vi "GLdrv_Read_USB.vi"(0 "hDevice":i32, 5 "Count":u32, 7 "Term(CrLf)":string="\r\n", 11 "error in (no error)":errorcluster, 12 "dwTimeOut":i32=1000) -> (4 "dup hDevice":i32, 6 "lpBuffer":string, 8 "lpNumberOfBytesRead":u32, 15 "error out":errorcluster)   [LabVIEW 2017]
uses:
  gtcusbr.dll
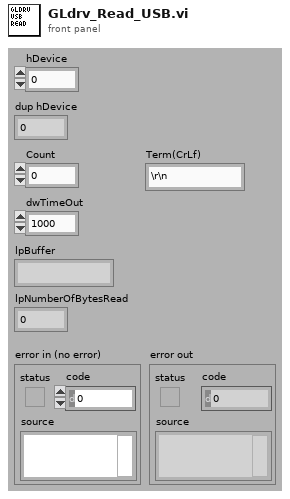
[diagram p1: front panel]
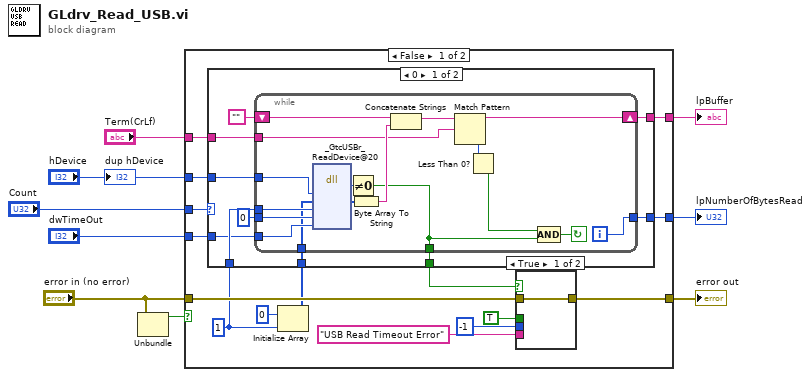
[diagram p0: block diagram]
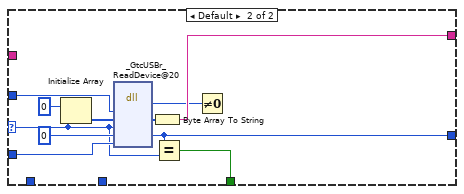
[diagram p2: hidden frame]
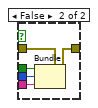
[diagram p3: hidden frame]
diagram:
  n1 = Unbundle("error in (no error)") -> ("status"=w4:bool)  [unwired: 2 out]
  n2 = case shown="FALSE" w4 {
    tunnel: "hDevice" -> [w24 _]
    tunnel: "dwTimeOut" -> [w23 _]
    tunnel: [w17 _] -> w7
    tunnel: [w16 _] -> w6
    tunnel: "error in (no error)" -> [w19 w69]
    tunnel: [w20 w69] -> w3
    tunnel: "Count" -> [w14 _]
    tunnel: "Term(CrLf)" -> [w10 _]
    frame False {
      w11 = 1 ("dimension size")
      n3 = Initialize Array(u8 0, w11) -> (w12:u8[])
      n4 = case shown="0" w14 {
        selector: w14 -> [_ w53]
        tunnel: w24 -> [w34 w62]
        tunnel: w23 -> [w26 w61]
        tunnel: [w31 w59] -> w17
        tunnel: [w30 w54] -> w16
        tunnel: [w29 w52] -> w15
        tunnel: w12 -> [w28 _]
        tunnel: w11 -> [w27 _]
        tunnel: w10 -> [w25 _]
        frame 0 {
          n5 = while {
            tunnel: w34 -> [w51]
            tunnel: w26 -> [w49]
            tunnel: [w39] -> w30
            shift-right: [w36] -> w31
            shift-left: "" -> [w46]
            tunnel: u32 0 ("lpNumberOfBytesRead") -> [w44]
            tunnel: w27 -> [w48]
            tunnel: [w40] -> w29
            tunnel: w28 -> [w41]
            tunnel: w25 -> [w35]
            i -> [w39]
            stop <- w42 continue-if-true
            n6 = dll-call lib="D:/src/LabVIEW/GL860/JP/LabView VI/Driver/gtcusbr.dll" fn="_GtcUSBr_ReadDevice@20"("hDevice"=w51, "lpBuffer"=w41, "nNumberOfBytesToRead"=w48, "lpNumberOfBytesRead"=w44, "dwTimeOut"=w49) -> ("BOOL"=w50:i8, "lpBuffer"=w47:u8[])  [unwired: 6 in, 3 out]
            n7 = Not Equal To 0?(x=w50) -> (x != 0?=w40:bool)
            n8 = Byte Array To String(unsigned byte array=w47) -> (string=w45:string)
            n9 = Concatenate Strings(w46, w45) -> (w38:string)
            n10 = Match Pattern(string=w38, regular expression=w35) -> (before substring=w36:string, offset past match=w43:i32)  [unwired: 3 out]
            n11 = Less Than 0?(x=w43) -> (x < 0?=w37:bool)
            n12 = Compound Arithmetic op=AND(w37, w40) -> (w42:bool)
          }
        }
        frame Default {
          n13 = Initialize Array(u8 0, w53) -> (w56:u8[])
          n14 = dll-call lib="D:/src/LabVIEW/GL860/JP/LabView VI/Driver/gtcusbr.dll" fn="_GtcUSBr_ReadDevice@20"("hDevice"=w62, "lpBuffer"=w56, "nNumberOfBytesToRead"=w53, "lpNumberOfBytesRead"=u32 0, "dwTimeOut"=w61) -> ("BOOL"=w58:i8, "lpBuffer"=w57:u8[], "lpNumberOfBytesRead"=w54:u32)  [unwired: 6 in, 2 out]
          n15 = Byte Array To String(unsigned byte array=w57) -> (string=w59:string)
          n16 = Equal?(x=w54, y=w53) -> (x = y?=w52:bool)
          n17 = Not Equal To 0?(x=w58) -> ()  [unwired: 1 out]
        }
      }
      n18 = case shown="TRUE" w15 {
        tunnel: [w63 w68] -> w20
        tunnel: w19 -> [w63 w67]
        tunnel: "USB Read Timeout Error" ("source") -> [_ w66]
        tunnel: -1 ("code") -> [_ w65]
        tunnel: TRUE ("status") -> [_ w64]
        frame True {
        }
        frame False {
          n19 = Bundle(cluster=w67, "status"=w64, "code"=w65, "source"=w66) -> (w68:errorcluster)
        }
      }
    }
    frame True {
    }
  }
  "lpBuffer" <- w7
  "lpNumberOfBytesRead" <- w6
  "error out" <- w3
  "dup hDevice" <- "hDevice"
